vi "Calc Limbus Correlation.vi"(6 "Y":u32, 8 "X":u32, 9 "Y_positions":i16[](array[numeric])=[0, 0, 0, 0, 0, 0, 0, 0, 0, 1, 1, 1, 1, 1, 1, 1, 1, 1, 1, 1, 1, 1, 1, 1, 1, 1, 1, 1, 1, 1, 1, 1, 1, 1, 1, 1, 1, 1, 1, 1, 1, 1, 0, 0, 0, 0, 0, 0, 0, 0, 0, 0, 0, 0, 0, 0, 0, 0, 0, 0, 0, 0, 0, 0, 0, 0, 0, 0, 0, 0, 0, 0, 0, 0, 0, 0, 0, 0, 0, 0, 0, 0, 0, 0, 0, 0, 0, 0, 0, 0, 0, 0, 0, 0, 0, 0, 0, 0, 0, 0], 10 "X_positions":i16[](array[numeric])=[1, 1, 1, 1, 1, 1, 1, 1, 1, 1, 1, 1, 1, 1, 1, 1, 1, 0, 0, 0, 0, 0, 0, 0, 0, 0, 0, 0, 0, 0, 0, 0, 0, 0, 0, 0, 0, 0, 0, 0, 0, 0, 0, 0, 0, 0, 0, 0, 0, 0, 0, 0, 0, 0, 0, 0, 0, 0, 0, 0, 0, 0, 0, 0, 0, 0, 0, 0, 0, 0, 0, 0, 0, 0, 0, 0, 0, 0, 0, 0, 0, 0, 0, 1, 1, 1, 1, 1, 1, 1, 1, 1, 1, 1, 1, 1, 1, 1, 1, 1], 11 "Picture":u8[][](array[numeric])) -> (3 "Grade":u32)   [LabVIEW 2015]
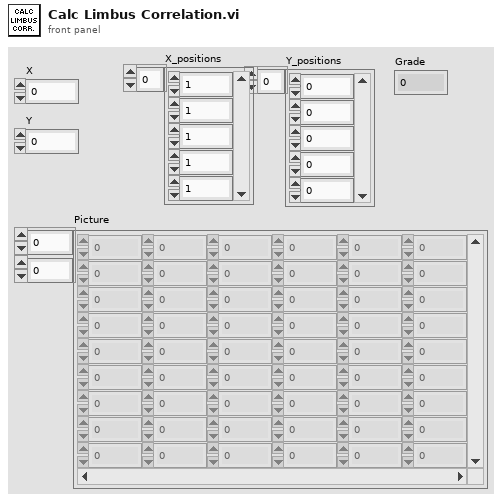
[diagram p1: front panel]
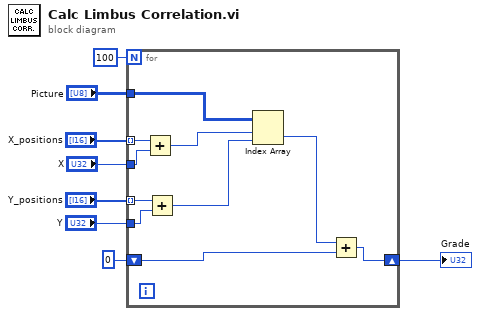
[diagram p0: block diagram]
diagram:
  n1 = for {
    N: 100 -> [_]
    tunnel: "Picture" -> [w18]
    tunnel: "X_positions" -> [w17] mode=indexing
    tunnel: "Y_positions" -> [w11] mode=indexing
    shift-right: [w14] -> w3
    shift-left: u32 0 -> [w15]
    tunnel: "X" -> [w12]
    tunnel: "Y" -> [w9]
    n2 = Add(x=w17, y=w12) -> (x+y=w13:u32)
    n3 = Add(x=w11, y=w9) -> (x+y=w10:u32)
    n4 = Index Array(array=w18, index (row)=w13, index (col)=w10) -> (element=w16:u8)
    n5 = Add(x=w16, y=w15) -> (x+y=w14:u32)
  }
  "Grade" <- w3
